vi "minicryo_T dependent RH sequence_202102.vi"() -> ()   [LabVIEW 2013]
uses:
  subVI/Global 2.vi
  subVI/DeltaRamp_globals.vi
  subVI/B_Globals.vi
panel:
  out "Output":path=path "C:/User Data/Guang/20210225 EuS10-V10-EuS20-Nb3 New/_T=1.75K.txt"
  in  "Sub":string
  in  "Directory":path=path "C:/User Data/Guang/20210225 EuS10-V10-EuS20-Nb3 New"
  in  "B_rate":dbl=0.05
  in  "B_max":dbl=0.05
  in  "Settle [Mins]":dbl=20.0
  in  "T Ramp Rate":dbl=0.20000000000000004
  in  "Temp":dbl[](array[numeric])=[1.65, 1.7, 1.75, 1.8, 1.85, 1.9, 1.95, 2.0, 2.5, 3.0, 4.0]
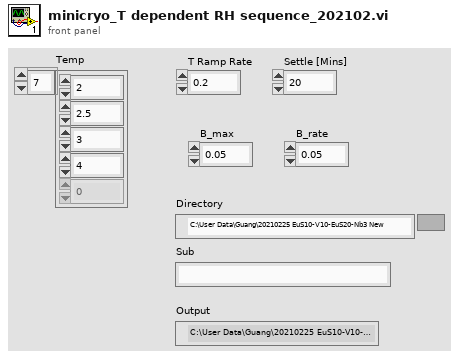
[diagram p1: front panel]
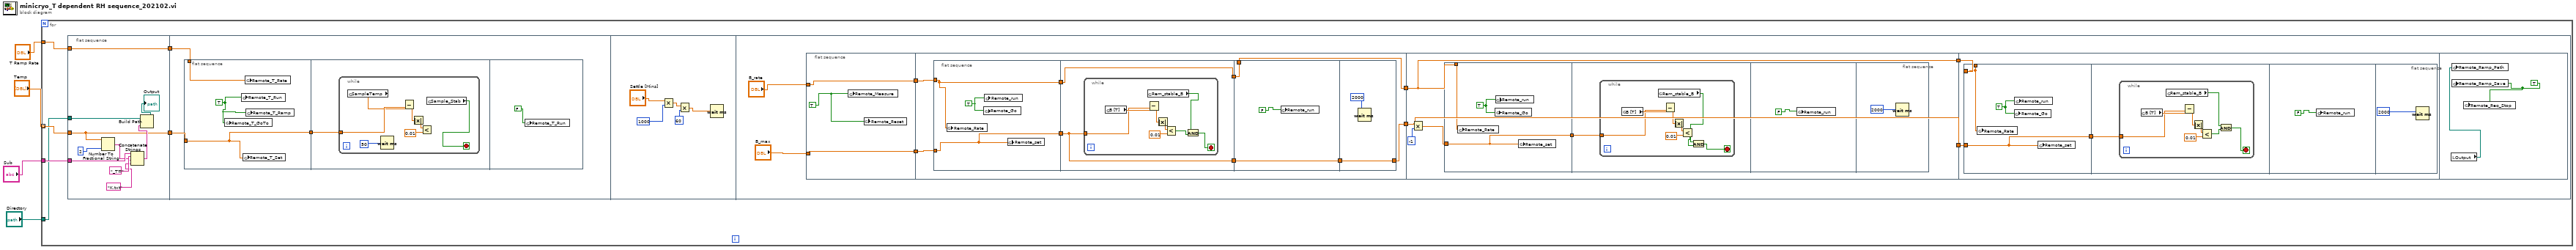
[diagram p0: block diagram]
diagram:
  n1 = for {
    tunnel: "Temp" -> [w10] mode=indexing
    tunnel: "T Ramp Rate" -> [w9]
    tunnel: "Directory" -> [w5]
    tunnel: "Sub" -> [w6]
    n2 = flat-sequence {
      tunnel: w9 -> [w20]
      tunnel: w10 -> [w11]
      tunnel: [w11] -> w8
      tunnel: [w20] -> w7
      tunnel: w6 -> [w19]
      tunnel: w5 -> [w16]
      tunnel: w8 -> [w22]
      tunnel: w7 -> [w21]
      frame #0 {
        n3 = Number To Fractional String(number=w11, precision (6)=2) -> (F-format string=w12:string)  [unwired: 2 in]
        n4 = Concatenate Strings(w19, "_T=", w12, "K.txt") -> (w14:string)
        n5 = Build Path(base path=w16, name or relative path=w14) -> (appended path=→"Output":path)
      }
      frame #1 {
        n6 = flat-sequence {
          tunnel: w22 -> [w25]
          tunnel: [w25] -> w23
          tunnel: w21 -> [w26]
          tunnel: w23 -> [w27]
          frame #0 {
            w24 = TRUE
            n7 = global write "Global 2.vi" "Remote_T_GoTo"(w24) -> ()
            n8 = global write "Global 2.vi" "Remote_T_Run"(w24) -> ()
            n9 = global write "Global 2.vi" "Remote_T_Set"(w25) -> ()
            n10 = global write "Global 2.vi" "Remote_T_Rate"(w26) -> ()
            n11 = global write "Global 2.vi" "Remote_T_Ramp"(w24) -> ()
          }
          frame #1 {
            n12 = while {
              tunnel: w27 -> [w34]
              stop <- w28 stop-if-true
              n13 = global read "Global 2.vi" "SampleTemp"() -> (w30:dbl)
              n14 = Wait (ms)(milliseconds to wait=50) -> ()  [unwired: 1 out]
              n15 = Subtract(x=w30, y=w34) -> (x-y=w33:dbl)
              n16 = Absolute Value(x=w33) -> (abs(x)=w32:dbl)
              n17 = Less?(x=w32, y=0.01) -> ()  [unwired: 1 out]
              n18 = global read "Global 2.vi" "Sample_Stab"() -> (w28:bool)
            }
          }
          frame #2 {
            n19 = global write "Global 2.vi" "Remote_T_Run"(FALSE) -> ()
          }
        }
      }
      frame #2 {
        n20 = Multiply(x="Settle [Mins]", y=1000) -> (x*y=w39:dbl)
        n21 = Multiply(x=w39, y=60) -> (x*y=w37:dbl)
        n22 = Wait (ms)(milliseconds to wait=w37) -> ()  [unwired: 1 out]
      }
      frame #3 {
        n23 = flat-sequence {
          tunnel: [w50] -> w44
          tunnel: "B_max" -> [w50]
          tunnel: "B_rate" -> [w49]
          tunnel: [w49] -> w41
          tunnel: [w55] -> w48
          tunnel: [w52] -> w47
          tunnel: w44 -> [w59]
          tunnel: w41 -> [w58]
          tunnel: w48 -> [w79]
          tunnel: w47 -> [w80]
          tunnel: [w80] -> w46
          tunnel: [w79] -> w45
          tunnel: w46 -> [w99]
          tunnel: w45 -> [w98]
          frame #0 {
            w51 = TRUE
            n24 = global write "DeltaRamp_globals.vi" "Remote_Measure"(w51) -> ()
            n25 = global write "DeltaRamp_globals.vi" "Remote_Reset"(w51) -> ()
          }
          frame #1 {
            n26 = flat-sequence {
              tunnel: [w62] -> w60
              tunnel: w59 -> [w62]
              tunnel: w58 -> [w61]
              tunnel: [w61] -> w53
              tunnel: w60 -> [w65]
              tunnel: [w65] -> w57
              tunnel: [w64] -> w54
              tunnel: w53 -> [w64]
              tunnel: w57 -> [w75]
              tunnel: [w75] -> w56
              tunnel: w54 -> [w74]
              tunnel: [w74] -> w52
              tunnel: [w77] -> w55
              tunnel: w56 -> [w77]
              frame #0 {
                w63 = TRUE
                n27 = global write "B_Globals.vi" "Remote_Rate"(w61) -> ()
                n28 = global write "B_Globals.vi" "Remote_Go"(w63) -> ()
                n29 = global write "B_Globals.vi" "Remote_run"(w63) -> ()
                n30 = global write "B_Globals.vi" "Remote_set"(w62) -> ()
              }
              frame #1 {
                n31 = while {
                  tunnel: w65 -> [w72]
                  stop <- w66 stop-if-true
                  n32 = global read "B_Globals.vi" "B [T]"() -> (w73:dbl)
                  n33 = global read "B_Globals.vi" "Rem_stable_B"() -> (w67:bool)
                  n34 = Subtract(x=w73, y=w72) -> (x-y=w71:dbl)
                  n35 = Absolute Value(x=w71) -> (abs(x)=w70:dbl)
                  n36 = Less?(x=w70, y=0.01) -> (x < y?=w68:bool)
                  n37 = And(x=w67, y=w68) -> (x .and. y?=w66:bool)
                }
              }
              frame #2 {
                n38 = global write "B_Globals.vi" "Remote_run"(FALSE) -> ()
              }
              frame #3 {
                n39 = Wait (ms)(milliseconds to wait=2000) -> ()  [unwired: 1 out]
              }
            }
          }
          frame #2 {
            n40 = Multiply(x=w79, y=-1) -> (x*y=w81:dbl)
            n41 = flat-sequence {
              tunnel: w81 -> [w84]
              tunnel: w80 -> [w85]
              tunnel: [w84] -> w83
              tunnel: w83 -> [w87]
              frame #0 {
                w86 = TRUE
                n42 = global write "B_Globals.vi" "Remote_Rate"(w85) -> ()
                n43 = global write "B_Globals.vi" "Remote_Go"(w86) -> ()
                n44 = global write "B_Globals.vi" "Remote_run"(w86) -> ()
                n45 = global write "B_Globals.vi" "Remote_set"(w84) -> ()
              }
              frame #1 {
                n46 = while {
                  tunnel: w87 -> [w94]
                  stop <- w88 stop-if-true
                  n47 = global read "B_Globals.vi" "B [T]"() -> (w95:dbl)
                  n48 = global read "B_Globals.vi" "Rem_stable_B"() -> (w90:bool)
                  n49 = Subtract(x=w95, y=w94) -> (x-y=w93:dbl)
                  n50 = Absolute Value(x=w93) -> (abs(x)=w92:dbl)
                  n51 = Less?(x=w92, y=0.01) -> (x < y?=w89:bool)
                  n52 = And(x=w90, y=w89) -> (x .and. y?=w88:bool)
                }
              }
              frame #2 {
                n53 = global write "B_Globals.vi" "Remote_run"(FALSE) -> ()
              }
              frame #3 {
                n54 = Wait (ms)(milliseconds to wait=2000) -> ()  [unwired: 1 out]
              }
            }
          }
          frame #3 {
            n55 = flat-sequence {
              tunnel: w98 -> [w102]
              tunnel: [w101] -> _
              tunnel: [w102] -> w100
              tunnel: w99 -> [w101]
              tunnel: w100 -> [w104]
              frame #0 {
                w103 = TRUE
                n56 = global write "B_Globals.vi" "Remote_Rate"(w101) -> ()
                n57 = global write "B_Globals.vi" "Remote_Go"(w103) -> ()
                n58 = global write "B_Globals.vi" "Remote_run"(w103) -> ()
                n59 = global write "B_Globals.vi" "Remote_set"(w102) -> ()
              }
              frame #1 {
                n60 = while {
                  tunnel: w104 -> [w111]
                  stop <- w106 stop-if-true
                  n61 = global read "B_Globals.vi" "B [T]"() -> (w112:dbl)
                  n62 = global read "B_Globals.vi" "Rem_stable_B"() -> (w105:bool)
                  n63 = Subtract(x=w112, y=w111) -> (x-y=w110:dbl)
                  n64 = Absolute Value(x=w110) -> (abs(x)=w109:dbl)
                  n65 = Less?(x=w109, y=0.01) -> (x < y?=w107:bool)
                  n66 = And(x=w105, y=w107) -> (x .and. y?=w106:bool)
                }
              }
              frame #2 {
                n67 = global write "B_Globals.vi" "Remote_run"(FALSE) -> ()
              }
              frame #3 {
                n68 = Wait (ms)(milliseconds to wait=2000) -> ()  [unwired: 1 out]
              }
            }
          }
          frame #4 {
            w116 = TRUE
            n69 = local read "Output"() -> (w115:path)
            n70 = global write "DeltaRamp_globals.vi" "Remote_Ramp_Path"(w115) -> ()
            n71 = global write "DeltaRamp_globals.vi" "Remote_Ramp_Save"(w116) -> ()
            n72 = global write "DeltaRamp_globals.vi" "Remote_Req_Stop"(w116) -> ()
          }
        }
      }
    }
  }
